vi "LVFunction_Imop_GetSoftwareConfig.vi"(0 "Configuration file path":path, 11 "error in":errorcluster) -> (4 "has_haso_soft":bool, 6 "has_casao_soft":bool, 8 "has_pharao_soft":bool, 10 "has_msqaure_soft":bool, 13 "error out":errorcluster, 14 "has_mtf_soft":bool, 15 "has_psf_soft":bool)   [LabVIEW 2020]
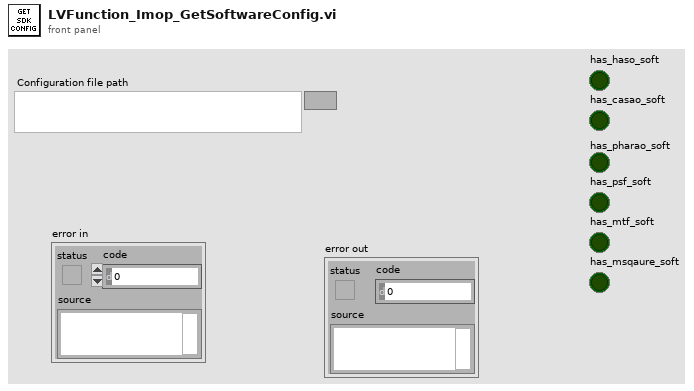
[diagram p1: front panel]
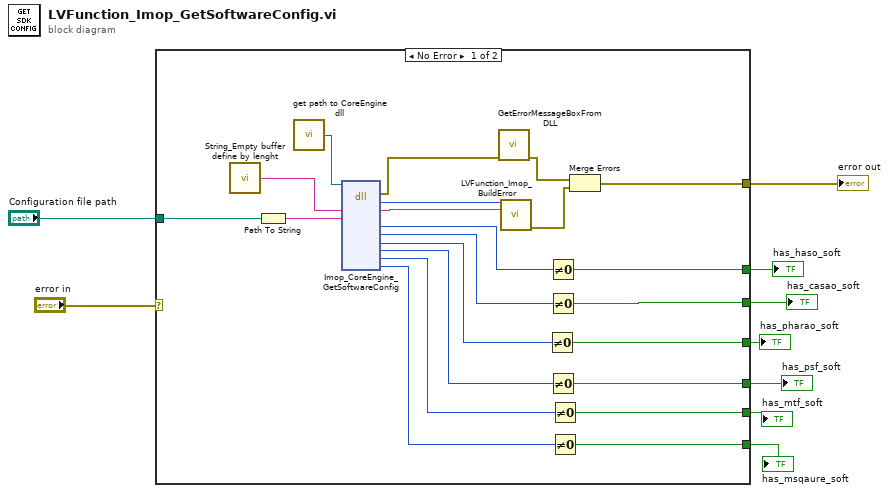
[diagram p0: block diagram]
diagram:
  n1 = case shown="No Error" "error in" {
    selector: "error in" -> [_ w32]
    tunnel: [w24 w32] -> w8
    tunnel: "Configuration file path" -> [w23 _]
    tunnel: [w16 _] -> w6
    tunnel: [w15 _] -> w5
    tunnel: [w14 _] -> w4
    tunnel: [w13 _] -> w3
    tunnel: [w12 _] -> w2
    tunnel: [w10 _] -> w1
    frame No Error {
      n2 = call "String_Empty buffer define by lenght.vi"() -> ("Empty buffer"=w25:string)  [unwired: 1 in]
      n3 = Path To String(path=w23) -> (string=w22:string)
      n4 = call "get path to CoreEngine dll.vi"() -> ("path to c_interface_vc100.dll"=w28:path)  [unwired: 12 in, 3 out]
      n5 = dll-call lib="D:/soft/HASO_v3/SVN_trunk/ImOpCoreEngine4_LV2011/DLLs/c_interface_vc100.dll" fn="Imop_CoreEngine_GetSoftwareConfig"(path in=w28, "message"=w25, "config_file_path"=w22) -> (error out=w29:errorcluster, "return type"=w27:i32, "message"=w26:string, "has_haso_sdk"=w21:u8, "has_casao_sdk"=w19:u8, "has_pharao_sdk"=w11:u8, "has_psf_sdk"=w20:u8, "has_mtf_sdk"=w18:u8, "has_msquare_sdk"=w17:u8)  [unwired: 9 in, 1 out]
      n6 = call "GetErrorMessageBoxFromDLL.vi"("error IN"=w29) -> ("error OUT"=w30:errorcluster)  [unwired: 10 in]
      n7 = call "LVFunction_Imop_BuildError.vi"("code"=w27, "String to Prepend to source (\"\")"=w26) -> ("error out"=w31:errorcluster)  [unwired: 13 in]
      n8 = Not Equal To 0?(x=w11) -> (x != 0?=w10:bool)
      n9 = Not Equal To 0?(x=w21) -> (x != 0?=w12:bool)
      n10 = Not Equal To 0?(x=w19) -> (x != 0?=w13:bool)
      n11 = Not Equal To 0?(x=w20) -> (x != 0?=w14:bool)
      n12 = Not Equal To 0?(x=w18) -> (x != 0?=w16:bool)
      n13 = Not Equal To 0?(x=w17) -> (x != 0?=w15:bool)
      n14 = Merge Errors(w30, w31) -> (w24:errorcluster)
    }
    frame Error {
    }
  }
  "error out" <- w8
  "has_mtf_soft" <- w6
  "has_msqaure_soft" <- w5
  "has_psf_soft" <- w4
  "has_casao_soft" <- w3
  "has_haso_soft" <- w2
  "has_pharao_soft" <- w1
